vi "Process.vi"(8 "error in (no error)":errorcluster, 10 "Pound in":refnum<class "Pound.lvclass">, 11 "Qbus in":refnum<class "Qbus.lvclass">) -> (0 "error out":errorcluster)   [LabVIEW 2017, in "EmsaDataEventCreator.lvlib"]
uses:
  <vilib>/addons/InsightCM/Devices/Shared/Emsa/EmsaDataEventCreator/EmsaDataEventCreator.lvlib
  <vilib>/addons/Qbus/Qbus.lvclass
  <vilib>/NI/Software Watchdog/Pound/Pound.lvclass
  <vilib>/addons/InsightCM/Devices/Shared/Emsa/EmsaDataEventCreator/controls/config.ctl
  <vilib>/addons/TraceLogger/TraceLogger.lvlib
  <vilib>/NI/Software Watchdog/Watchdog/Watchdog.lvclass
  <vilib>/addons/InsightCM/Devices/Shared/Common/DataFlow/DataFlow.lvlib
  <vilib>/addons/InsightCM/Devices/Shared/Common/DataEventCreator/DataEventCreator.lvlib
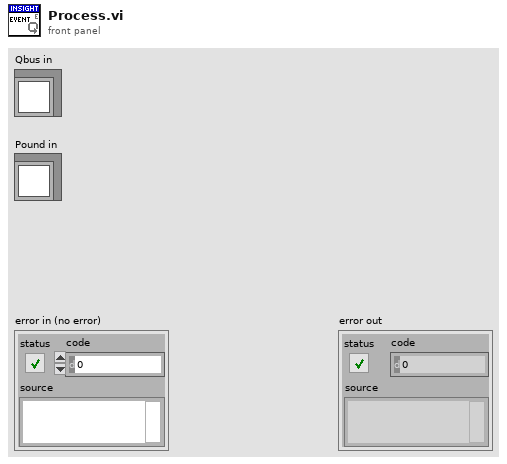
[diagram p1: front panel]
types:
  T1 = typedef "EmsaDataEventCreator.lvlib/config.ctl" = cluster{"DeviceName":string, "Registry":variant, "Sweep Params":variant}
  T2 = typedef "EmsaDataEventCreator.lvlib/RegisterSweepRoutedMessage.ctl" = cluster{"Group":string, "Sweeps":T3[]}
  T3 = typedef "EmsaDataEventCreator.lvlib/Registry_Sweep.ctl" = cluster{"Name":string, "DataSetType":T4, "Properties":T5[]}
  T4 = typedef "DataEvent.lvlib/DataSetType.ctl" = enum16{"Waveform", "SpeedProfile", "ThermalImage", "EmsaSweep"}
  T5 = typedef "KeyValuePair.ctl" = cluster{"Key":string, "Value":string}
  T6 = typedef "DataEventCreator.lvlib/RegisterTrendPoints.ctl" = cluster{"DataGroup":string, "Trends":T7[]}
  T7 = typedef "DataEventCreator.lvlib/Registry_Trend.ctl" = cluster{"TrendPointId":string, "DataSetName":string, "HighRate":bool, "Always Send":bool}
  T8 = typedef "DataFlow.lvlib/Data.ctl" = cluster{"DataGroup":string, "Waveforms":T9, "Map":T10, "Type":T11}
  T9 = typedef "wfmSGL_DVR.ctl" = refnum<data-value>
  T10 = typedef "PointValueMap.lvlib/PointMap.ctl" = refnum<data-value>
  T11 = typedef "DataFlow.lvlib/Type.ctl" = enum16{"High Rate", "Low Rate", "Burst Mode"}
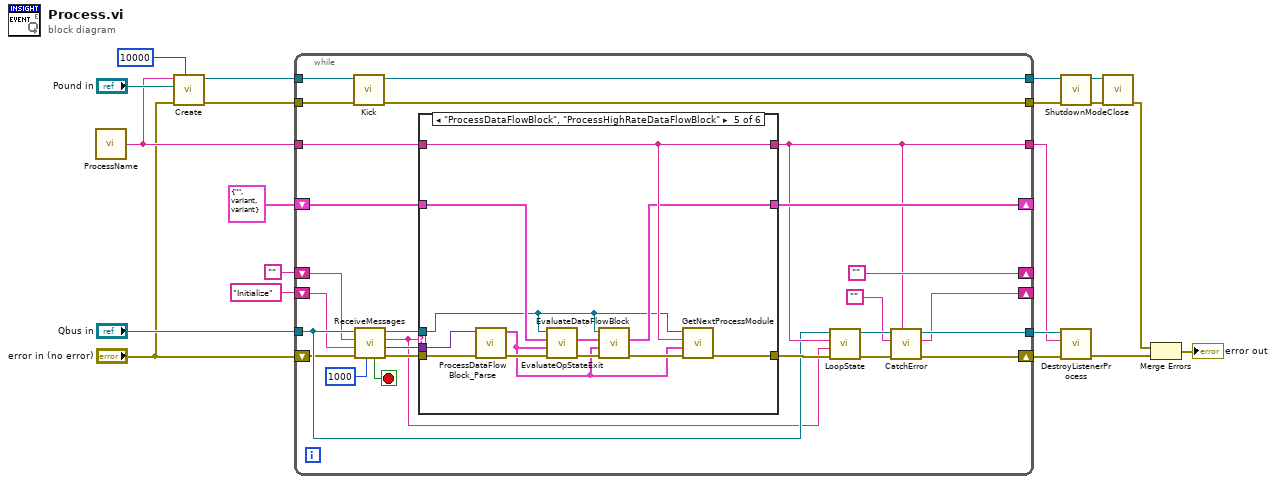
[diagram p0: block diagram]
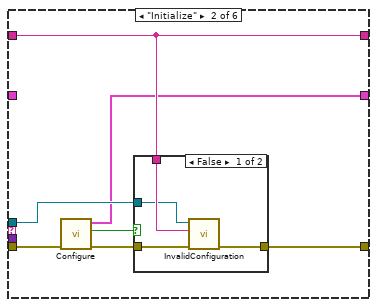
[diagram p3: hidden frame]
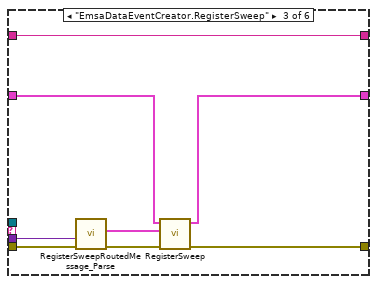
[diagram p5: hidden frame]
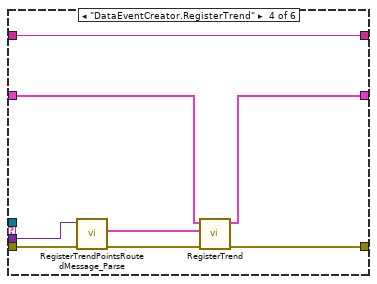
[diagram p6: hidden frame]
diagram:
  n1 = call <vilib>:"ProcessName.vi"() -> ("process name"=w4:string)  [unwired: 5 in]
  n2 = call <vilib>:"Create.vi"("Execution Timeout (ms)"=u32 10000, "error in (no error)"="error in (no error)", "Pound"="Pound in", "Name"=w4) -> ("error out"=w9:errorcluster, "Watchdog"=w15:refnum<data-value>)  [unwired: 6 in]
  n3 = while {
    shift-right: [""] -> _
    shift-left: "" -> [w29]
    tunnel: "Qbus in" -> [w30]
    tunnel: w4 -> [w33]
    tunnel: [w42] -> w18
    tunnel: [w32] -> w17
    shift-right: [w41] -> _
    shift-left: "Initialize" -> [w28]
    shift-right: [w44] -> _
    shift-left: T1 {"DeviceName"="", "Registry"=variant, "Sweep Params"=variant} ("config") -> [w45]
    tunnel: w15 -> [w39]
    tunnel: [w38] -> w11
    tunnel: w9 -> [w37]
    tunnel: [w36] -> w8
    shift-right: [w43] -> w19
    shift-left: "error in (no error)" -> [w27]
    stop <- w25 stop-if-true
    n4 = call <vilib>:"Kick.vi"("error in (no error)"=w37, "Watchdog"=w39) -> ("error out"=w36:errorcluster, "Watchdog"=w38:refnum<data-value>)  [unwired: 8 in]
    n5 = call <vilib>:"ReceiveMessages.vi"("Timeout(1000)"=1000 ("milliseconds to wait"), "error in (no error)"=w27, "priority action"=w28, "default action"=w29, "Qbus in"=w30) -> ("error out"=w24:errorcluster, "message value"=w23:variant, "action"=w22:string, "Qbus out"=w21:refnum<class "Qbus.lvclass">, "exit"=w25:bool)  [unwired: 2 in]
    n6 = case shown="\"ProcessDataFlowBlock\", \"ProcessHighRateDataFlowBlock\"" w22 {
      tunnel: w24 -> [w47 w53 w67 w76 w88 w92]
      tunnel: w21 -> [_ w54 _ _ w79 _]
      tunnel: [w47 w56 w64 w70 w87 w92] -> w40
      tunnel: w23 -> [_ _ w68 w75 w89 _]
      tunnel: w45 -> [w49 _ w63 w72 w85 w91]
      tunnel: [w49 w51 w62 w71 w81 w91] -> w44
      tunnel: [w48 w55 w69 w77 w86 w90] -> w32
      tunnel: w33 -> [w48 w55 w69 w77 w86 w90]
      frame "", Default {
      }
      frame "Initialize" {
        n7 = call <vilib>:"Configure.vi"("error in (no error)"=w53) -> ("error out"=w52:errorcluster, "valid configuration"=w50:bool, "config out"=w51:T1)  [unwired: 8 in]
        n8 = case shown="False" w50 {
          tunnel: w52 -> [w57 w61]
          tunnel: [w60 w61] -> w56
          tunnel: w54 -> [w58 _]
          tunnel: w55 -> [w59 _]
          frame False {
            n9 = call <vilib>:"InvalidConfiguration.vi"("error in (no error)"=w57, "description"=w59, "Qbus in"=w58) -> ("error out"=w60:errorcluster)  [unwired: 7 in, 1 out]
          }
          frame True {
            # "Valid configuration"
          }
        }
      }
      frame "EmsaDataEventCreator.RegisterSweep" {
        n10 = call <vilib>:"RegisterSweepRoutedMessage_Parse.vi"("error in (no error)"=w67, "message"=w68) -> ("error out"=w65:errorcluster, "register sweep routed message"=w66:T2)  [unwired: 8 in]
        n11 = call <vilib>:"RegisterSweep.vi"("error in"=w65, "RegisterSweepRoutedMessage"=w66, "config"=w63) -> ("error out"=w64:errorcluster, "config out"=w62:T1)  [unwired: 7 in]
      }
      frame "DataEventCreator.RegisterTrend" {
        n12 = call <vilib>:"RegisterTrendPointsRoutedMessage_Parse.vi"("error in (no error)"=w76, "message"=w75) -> ("error out"=w74:errorcluster, "RegisterTrend"=w73:T6)  [unwired: 8 in]
        n13 = call <vilib>:"RegisterTrend.vi"("error in"=w74, "RegisterTrend"=w73, "config"=w72) -> ("error out"=w70:errorcluster, "config out"=w71:T1)  [unwired: 7 in]
      }
      frame "ProcessDataFlowBlock", "ProcessHighRateDataFlowBlock" {
        n14 = call <vilib>:"ProcessDataFlowBlock_Parse.vi"("error in (no error)"=w88, "body"=w89) -> ("error out"=w83:errorcluster, "data"=w80:T8)  [unwired: 8 in]
        n15 = call <vilib>:"EvaluateOpStateExit.vi"("error in (no error)"=w83, "data flow"=w80, "config"=w85, "Qbus in"=w79) -> ("error out"=w84:errorcluster, "config out"=w78:T1)  [unwired: 6 in]
        n16 = call <vilib>:"EvaluateDataFlowBlock.vi"("error in (no error)"=w84, "data"=w80, "config"=w78, "Qbus"=w79) -> ("error out"=w82:errorcluster, "config out"=w81:T1)  [unwired: 6 in]
        n17 = call <vilib>:"GetNextProcessModule.vi"("error in (no error)"=w82, "data"=w80, "source"=w86, "Qbus in"=w79) -> ("error out"=w87:errorcluster)  [unwired: 6 in, 1 out]
      }
      frame "Exit" {
      }
    }
    n18 = call <vilib>:"LoopState.vi"("error in (no error)"=w40, "loop action"=w22, "process name"=w32, "Qbus in"=w30) -> ("error out"=w35:errorcluster, "Qbus out"=w34:refnum<class "Qbus.lvclass">)  [unwired: 6 in]
    n19 = call <vilib>:"CatchError.vi"("source"=w32, "error in (no error)"=w35, "next action in"="", "Qbus in"=w34) -> ("error out"=w43:errorcluster, "next action out"=w41:string, "Qbus out"=w42:refnum<class "Qbus.lvclass">)  [unwired: 5 in]
  }
  n20 = call <vilib>:"ShutdownMode.vi"("error in (no error)"=w8, "Watchdog"=w11) -> ("error out"=w10:errorcluster, "Watchdog"=w12:refnum<data-value>)  [unwired: 8 in]
  n21 = call <vilib>:"DestroyListenerProcess.vi"("error in (no error)"=w19, "process name"=w17, "Qbus in"=w18) -> ("error in (no error)"=w7:errorcluster)  [unwired: 7 in, 1 out]
  n22 = call <vilib>:"Close.vi"("error in (no error)"=w10, "Watchdog"=w12) -> ("error out"=w6:errorcluster)  [unwired: 9 in]
  n23 = Merge Errors(w6, w7) -> (→"error out":errorcluster)
